vi "Cleanup.vi"(8 "error in (no error)":errorcluster, 11 "Dashboard Panel in":refnum<class "Dashboard Panel.lvclass">) -> (0 "error out":errorcluster)   [LabVIEW 2020, in "SB App.lvlib" / "Dashboard Panel.lvclass"]
uses:
  Dashboard Panel.lvclass
  Dashboard Panel.lvclass/Dashboard Panel.ctl
  <vilib>/IlluminatedG/IG OOPanel/OOPanel/Panel/Panel.lvclass
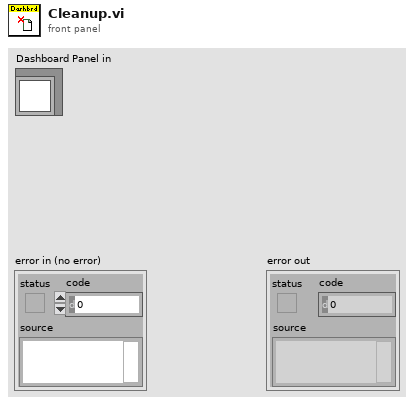
[diagram p1: front panel]
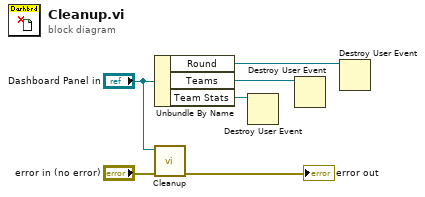
[diagram p0: block diagram]
diagram:
  n1 = Unbundle By Name("Dashboard Panel in") -> ("Round"=w1:refnum<user-event>, "Teams"=w2:refnum<user-event>, "Team Stats"=w3:refnum<user-event>)
  n2 = call-parent "Cleanup.vi"("error in (no error)"="error in (no error)", "Panel in"="Dashboard Panel in") -> ("error out"=→"error out":errorcluster)  [unwired: 9 in]
  n3 = Destroy User Event(user event=w3) -> ()  [unwired: 1 in, 1 out]
  n4 = Destroy User Event(user event=w2) -> ()  [unwired: 1 in, 1 out]
  n5 = Destroy User Event(user event=w1) -> ()  [unwired: 1 in, 1 out]
